vi "generateEventSummaryState.vi"(8 "error in (no error)":errorcluster, 10 "EventSummaryState":T1, 11 "UserEvents in":refnum<class "UserEvents.lvclass">) -> (0 "error out":errorcluster, 3 "UserEvents out":refnum<class "UserEvents.lvclass">)   [LabVIEW 2016, in "UserEvents.lvclass"]
uses:
  UserEvents.lvclass
  DataTypes/Topics/EventSummaryState.ctl
  DataTypes/Topics/Parts/Timestamp.ctl
  DataTypes/Topics/Parts/SummaryStates.ctl
  UserEvents.lvclass/UserEvents.ctl
  DataTypes/Topics/M1M3SupportTopics.lvlib
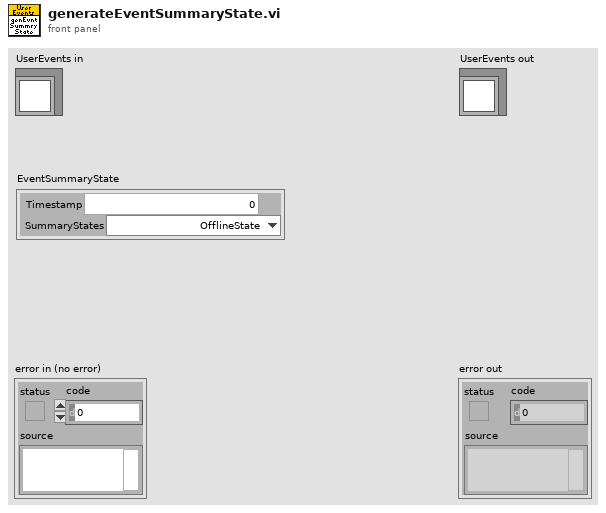
[diagram p1: front panel]
types:
  T1 = typedef "M1M3SupportTopics.lvlib/EventSummaryState.ctl" = cluster{"Timestamp":T2, "SummaryStates":T3}
  T2 = typedef "M1M3SupportTopics.lvlib/Timestamp.ctl" = dbl
  T3 = typedef "M1M3SupportTopics.lvlib/SummaryStates.ctl" = enum16{"OfflineState", "StandbyState", "DisabledState", "EnabledState", "FaultState"}
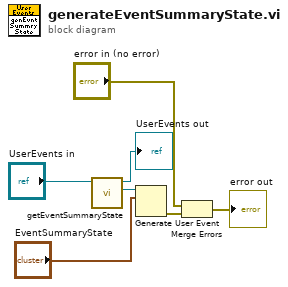
[diagram p0: block diagram]
diagram:
  n1 = call "getEventSummaryState.vi"("UserEvents in"="UserEvents in") -> ("EventSummaryState"=w7:refnum<user-event>, "UserEvents out"=→"UserEvents out":refnum<class "UserEvents.lvclass">)  [unwired: 9 in]
  n2 = Generate User Event(user event=w7, event data cluster="EventSummaryState") -> (error out=w3:errorcluster)  [unwired: 2 in, 1 out]
  n3 = Merge Errors("error in (no error)", w3) -> (→"error out":errorcluster)
